vi "Cancel Current Operation.vi"(8 "error in (no error)":errorcluster, 11 "Application in":refnum<class "Application.lvclass">) -> (0 "error out":errorcluster, 3 "Application out":refnum<class "Application.lvclass">)   [LabVIEW 2023, in "Application.lvlib" / "Application.lvclass"]
uses:
  Application.lvclass
  Mode.ctl
  Application.lvclass/Application.ctl
  Application.lvlib
panel:
  in  "New Mode":T1=enum."Cancel"
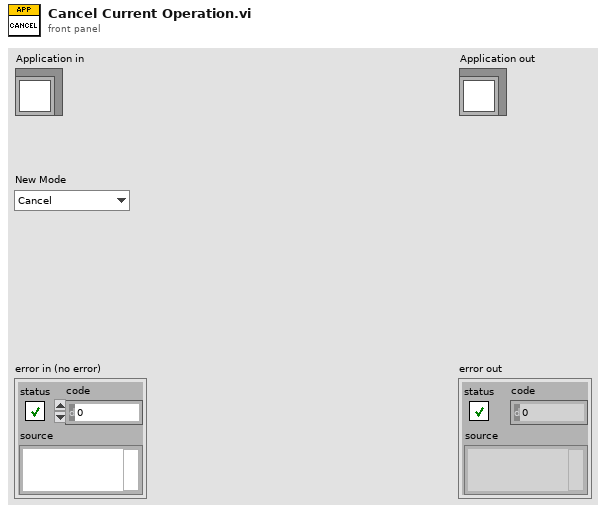
[diagram p1: front panel]
types:
  T1 = typedef "Application.lvlib/Mode.ctl" = enum16{"Idle", "Cancel", "Live", "Stream", "Autofocus", "Z-Stack"}
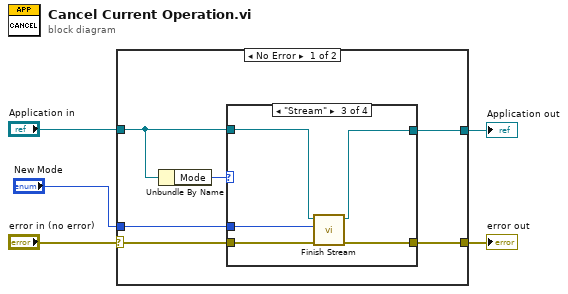
[diagram p0: block diagram]
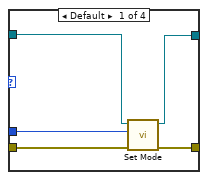
[diagram p2: hidden frame]
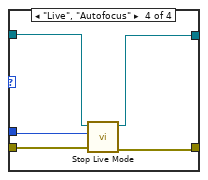
[diagram p4: hidden frame]
diagram:
  n1 = case shown="No Error" "error in (no error)" {
    selector: "error in (no error)" -> [w9 w30]
    tunnel: [w10 w30] -> w4
    tunnel: [w11 w29] -> w2
    tunnel: "Application in" -> [w8 w29]
    tunnel: "New Mode" -> [w6 _]
    frame No Error {
      n2 = Unbundle By Name(w8) -> ("Mode"=w7:T1)
      n3 = case shown="\"Stream\"" w7 {
        tunnel: [w14 w18 w23 w26] -> w11
        tunnel: [w15 w17 w22 w27] -> w10
        tunnel: w8 -> [w13 w18 w20 w25]
        tunnel: w9 -> [w16 w17 w21 w28]
        tunnel: w6 -> [w12 _ w19 w24]
        frame Default {
          n4 = call-dynamic "Set Mode.vi"("error in (no error)"=w16, "New Mode"=w12, "Application in"=w13) -> ("error out"=w15:errorcluster, "Application out"=w14:refnum<class "Application.lvclass">)  [unwired: 7 in]
        }
        frame "Idle" {
        }
        frame "Stream" {
          n5 = call-dynamic "Finish Stream.vi"("error in (no error)"=w21, "New Mode"=w19, "Application in"=w20) -> ("error out"=w22:errorcluster, "Application out"=w23:refnum<class "Application.lvclass">)  [unwired: 7 in]
        }
        frame "Live", "Autofocus" {
          n6 = call-dynamic "Stop Live Mode.vi"("error in (no error)"=w28, "Mode"=w24, "Application in"=w25) -> ("error out"=w27:errorcluster, "Application out"=w26:refnum<class "Application.lvclass">)  [unwired: 7 in]
        }
      }
    }
    frame Error {
    }
  }
  "error out" <- w4
  "Application out" <- w2
